vi "runTimestampTest.vi"() -> ()   [LabVIEW 2016]
uses:
  <vilib>/rvi/interface/nirviOpenFPGA/nirviOpenFPGA.xnode
  <vilib>/rvi/interface/nirviMethod/nirviMethod.xnode
  <vilib>/FPGAPlugInAG/Dynamic/niLvFpga_Abort_Dynamic.vi
  <vilib>/FPGAPlugInAG/Dynamic/niLvFpga_Reset_Dynamic.vi
  <vilib>/FPGAPlugInAG/Dynamic/niLvFpga_Run_Dynamic.vi
  <vilib>/rvi/errors/niLvFpgaMergeErrorWithErrorCode.vi
  <vilib>/rvi/interface/nirviCloseFPGA/nirviCloseFPGA.xnode
  FPGA Bitfiles/Modbus_FPGATarget_timestampTest_bycwkAQVPHw.lvbitx
  <vilib>/FPGAPlugInAG/cRIO-9038/niLvFpga_Open_cRIO-9038.vi
  <vilib>/rvi/interface/common/dynamic/niFpgaDynamicAddResources.vi
  <vilib>/FPGAPlugInAG/Dynamic/niLvFpga_ReadFifo_Dynamic.vi
  <vilib>/FPGAPlugInAG/Dynamic/niLvFpga_WriteFifo_Dynamic.vi
  <vilib>/FPGAPlugInAG/Dynamic/niLvFpga_Close_Dynamic.vi
panel:
  out "Avg Error":dbl
  out "Min Error":i64
  out "Max Error":i64
  out "Long Term Chart":dbl(graph)
  out "Short Term Chart":i64(graph)
  out "Error":i64
  out "FPGATime":u64
  out "RTTime":u64
  in  "Boolean":bool
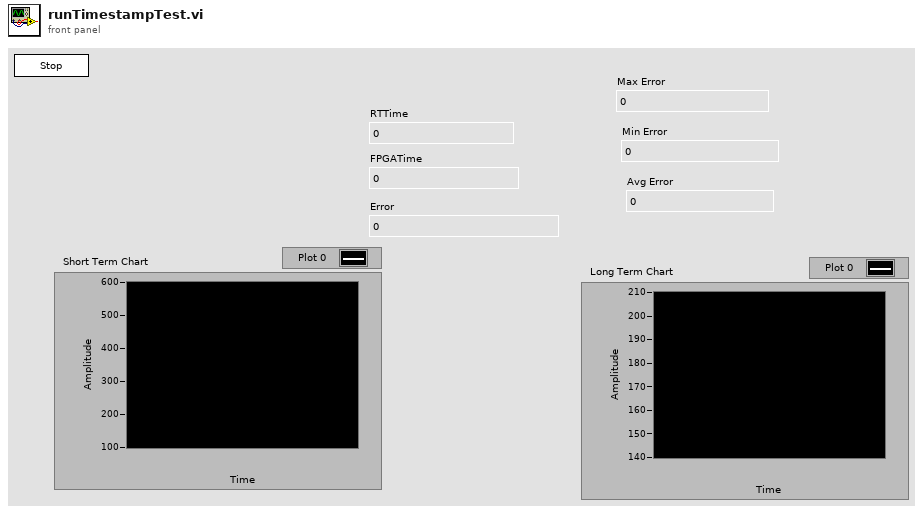
[diagram p1: front panel]
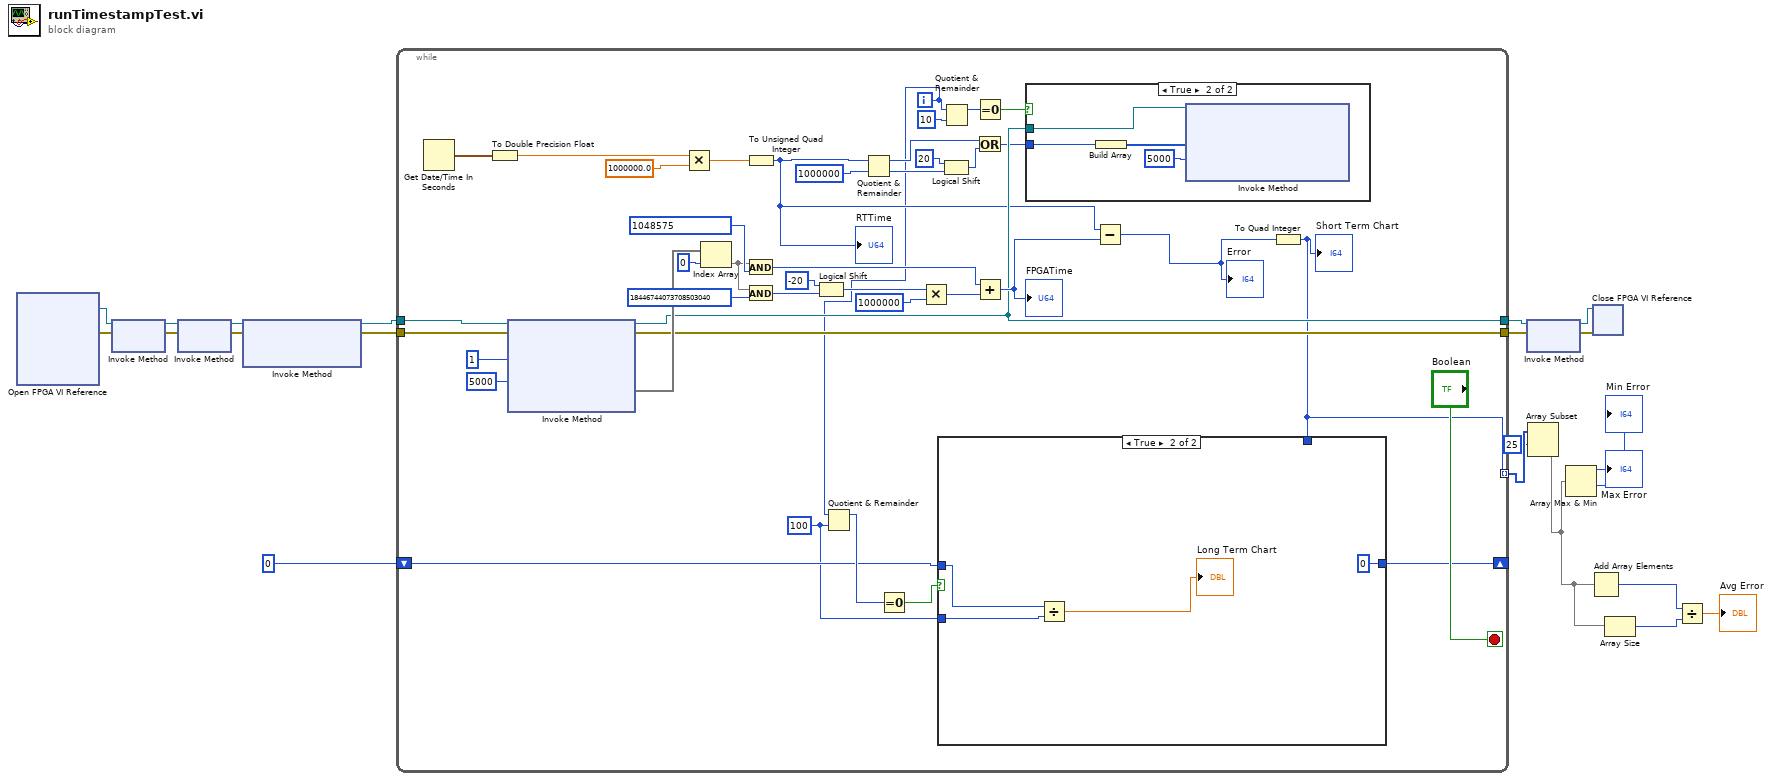
[diagram p0: block diagram]
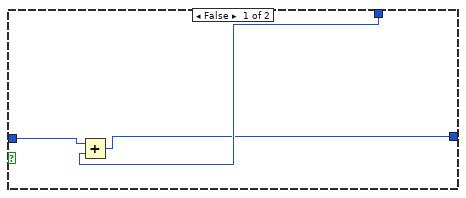
[diagram p2: hidden frame]
diagram:
  n1 = xnode "Open FPGA VI Reference"() -> ("FPGA VI Reference Out"=w21:refnum<k20>, "error out"=w20:errorcluster)  [unwired: 2 in]
  n2 = xnode "Invoke Method"("FPGA VI Reference In"=w21, "error in"=w20) -> ("FPGA VI Reference Out"=w19:refnum<k20>, "error out"=w18:errorcluster)
  n3 = xnode "Invoke Method"("FPGA VI Reference In"=w19, "error in"=w18) -> ("FPGA VI Reference Out"=w17:refnum<k20>, "error out"=w16:errorcluster)
  n4 = xnode "Invoke Method"("FPGA VI Reference In"=w17, "error in"=w16) -> ("FPGA VI Reference Out"=w15:refnum<k20>, "error out"=w13:errorcluster)  [unwired: 1 in]
  n5 = while {
    tunnel: w15 -> [w61]
    tunnel: [w41] -> w14
    tunnel: w13 -> [w56]
    tunnel: [w55] -> w12
    shift-right: [w24] -> _
    shift-left: i64 0 -> [w25]
    tunnel: [w22] -> w3 mode=indexing
    i -> [w26]
    stop <- "Boolean" stop-if-true
    w23 = 100 ("y")
    n6 = Get Date/Time In Seconds() -> (seconds since 1Jan1904=w34:timestamp)
    n7 = To Double Precision Float(number=w34) -> (double precision float=w33:dbl)
    n8 = xnode "Invoke Method"("FPGA VI Reference In"=w61, "error in"=w56, "Number of Elements"=u32 1, "Timeout (ms)"=5000) -> ("FPGA VI Reference Out"=w41:refnum<k20>, "error out"=w55:errorcluster, "Data"=w58:void[])  [unwired: 1 out]
    n9 = Multiply(x=w33, y=1000000.0) -> (x*y=w31:dbl)
    n10 = Index Array(array=w58, index=0) -> (element=w52)
    n11 = To Unsigned Quad Integer(1:w31) -> (0:w30:u64)
    "RTTime" <- w30
    n12 = And(x=w52, y=u64 1048575) -> (x .and. y?=w47:u64)
    n13 = And(x=w52, y=u64 18446744073708503040) -> (x .and. y?=w51:u64)
    n14 = Logical Shift(y=i16 -20, x=w51) -> (x << y=w49:u64)
    n15 = Quotient & Remainder(x=w26, y=w23) -> (x-y*floor(x/y)=w28:i32)  [unwired: 1 out]
    n16 = Quotient & Remainder(x=w30, y=u64 1000000) -> (x-y*floor(x/y)=w40:u64, floor(x/y)=w37:u64)
    n17 = Equal To 0?(x=w28) -> (x = 0?=w27:bool)
    n18 = Multiply(x=w49, y=u64 1000000) -> (x*y=w46:u64)
    n19 = Logical Shift(y=i16 20, x=w37) -> (x << y=w39:u64)
    n20 = Quotient & Remainder(x=w26, y=10) -> (x-y*floor(x/y)=w43:i32)  [unwired: 1 out]
    n21 = Equal To 0?(x=w43) -> (x = 0?=w42:bool)
    n22 = Or(x=w40, y=w39) -> (x .or. y?=w35:u64)
    n23 = Add(x=w47, y=w46) -> (x+y=w45:u64)
    "FPGATime" <- w45
    n24 = case shown="True" w42 {
      tunnel: w41 -> [_ w73]
      tunnel: w35 -> [_ w71]
      frame False {
      }
      frame True {
        n25 = Build Array(w71) -> (w70:u64[])
        n26 = xnode "Invoke Method"("FPGA VI Reference In"=w73, "Data"=w70, "Timeout (ms)"=5000) -> ()  [unwired: 1 in, 3 out]
      }
    }
    n27 = Subtract(x=w30, y=w45) -> (x-y=w29:u64)
    "Error" <- w29
    n28 = To Quad Integer(1:w29) -> (0:w22:i64)
    "Short Term Chart" <- w22
    n29 = case shown="True" w27 {
      tunnel: w22 -> [w64 _]
      tunnel: w25 -> [w65 w69]
      tunnel: [w63 i64 0] -> w24
      tunnel: w23 -> [_ w68]
      frame False {
        n30 = Add(x=w65, y=w64) -> (x+y=w63:i64)
      }
      frame True {
        n31 = Divide(x=w69, y=w68) -> (x/y=→"Long Term Chart":dbl)
      }
    }
  }
  n32 = xnode "Invoke Method"("FPGA VI Reference In"=w14, "error in"=w12) -> ("FPGA VI Reference Out"=w11:refnum<k20>, "error out"=w10:errorcluster)
  n33 = Array Subset(array=w3, index=25) -> (w1:i64[])  [unwired: 1 in]
  n34 = Array Max & Min(array=w1) -> (max value=→"Max Error":i64, min value=→"Min Error":i64)  [unwired: 2 out]
  n35 = Add Array Elements(numeric array=w1) -> (sum=w6:i64)
  n36 = xnode "Close FPGA VI Reference"("FPGA VI Reference In"=w11, "error in"=w10) -> ()  [unwired: 1 out]
  n37 = Array Size(array=w1) -> (size(s)=w5:i32)
  n38 = Divide(x=w6, y=w5) -> (x/y=→"Avg Error":dbl)
